vi "SubVI_Arrow.vi"(11 "ScanCode":i16) -> (3 "Arrow key":bool)   [LabVIEW 2016]
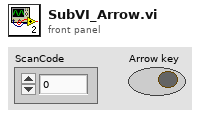
[diagram p1: front panel]
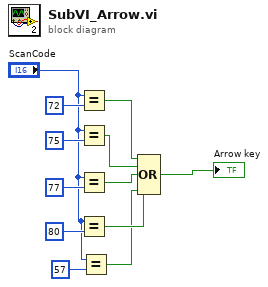
[diagram p0: block diagram]
diagram:
  n1 = Equal?(x="ScanCode", y=i16 72) -> (x = y?=w8:bool)
  n2 = Equal?(x="ScanCode", y=i16 75) -> (x = y?=w7:bool)
  n3 = Equal?(x="ScanCode", y=i16 77) -> (x = y?=w6:bool)
  n4 = Equal?(x="ScanCode", y=i16 80) -> (x = y?=w4:bool)
  n5 = Equal?(x="ScanCode", y=i16 57) -> (x = y?=w3:bool)
  n6 = Compound Arithmetic op=OR(w8, w7, w6, w4, w3) -> (→"Arrow key":bool)
